vi "Execute.vi"(8 "error in":errorcluster, 11 "Change PAS Flow in":refnum<class "Change PAS Flow.lvclass">) -> (0 "error out":errorcluster, 1 "Next Step?":bool, 2 "MSG":string, 3 "Change PAS Flow out":refnum<class "Change PAS Flow.lvclass">)   [LabVIEW 2015, in "Change PAS Flow.lvclass"]
uses:
  Change PAS Flow.lvclass
  Reusable/Sequence/STEPS/LEAVES/Double/Switch DBL.lvclass/Switch DBL.ctl
  Reusable/Sequence/STEPS/LEAVES/Double/Read val.vi
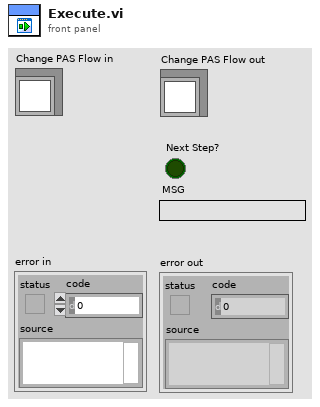
[diagram p1: front panel]
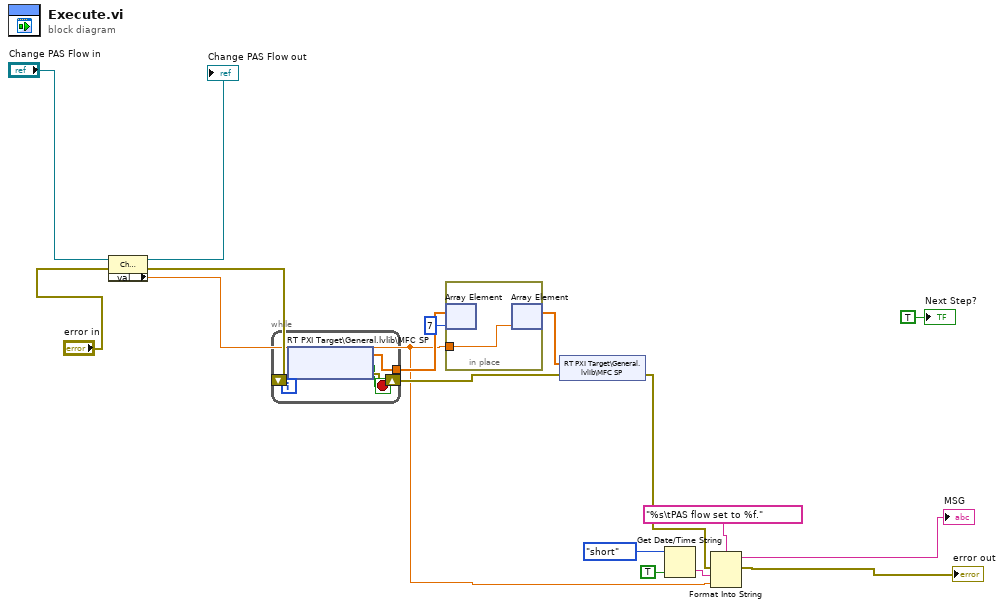
[diagram p0: block diagram]
diagram:
  n1 = property class="Change PAS Flow.lvclass"(reference="Change PAS Flow in", error in="error in") -> (reference out=→"Change PAS Flow out":refnum<class "Change PAS Flow.lvclass">, error out=w8:errorcluster, "val"=w7:dbl)
  n2 = while {
    tunnel: [w20] -> w16
    shift-right: [w21] -> w17
    shift-left: w8 -> [w19]
    stop <- w18 stop-if-true
    n3 = shared-variable "RT PXI Target\\General.lvlib\\MFC SP"(error in=w19) -> (w20:sgl[], error out=w21:errorcluster, w18:bool)  [unwired: 1 in]
  }
  n4 = in-place {
    in-place-border: w7 -> [w22]
    n5 = in-place-array #1(w16, 7) -> ()  [unwired: 1 out]
    n6 = in-place-array #1(w22) -> (w15:sgl[])  [unwired: 1 out]
  }
  n7 = shared-variable "RT PXI Target\\General.lvlib\\MFC SP"(w15, error in=w17) -> (error out=w6:errorcluster)
  n8 = Get Date/Time String(date format (0)=enum16{"short", "long", "abbreviated"}."short", want seconds? (F)=TRUE) -> (time string=w12:string)  [unwired: 1 in, 1 out]
  n9 = Format Into String(format string="%s\tPAS flow set to %f.", error in=w6, w12, w7) -> (resulting string=→"MSG":string, error out=→"error out":errorcluster)  [unwired: 1 in]
  "Next Step?" <- TRUE ("Next Step?")
